vi "Test Pincer Ctrl.vi"() -> ()   [LabVIEW 2010]
uses:
  <vilib>/platform/TimedLoop/XDataNode/XDataNode.xnode
  <vilib>/Platform/TimedLoop/XDataNode/nitl_modes.ctl
  <vilib>/Platform/TimedLoop/XDataNode/XDNodeRunTimeDep.lvlib
  <vilib>/Platform/TimedLoop/XDataNode/wakeup.ctl
  <vilib>/Platform/TimedLoop/XDataNode/timing_clust.ctl
  <vilib>/rvi/interface/nirviReadWriteControl/nirviReadWriteControl.xnode
  FPGA Bitfiles/IRISSControl_FPGATarget_IRISSFPGAIOv3.3_r-h2UkgnQFc.lvbitx
  IRISS_FPGA_IO_v3.3.vi
  <vilib>/rvi/interface/nirviOpenFPGA/nirviOpenFPGA.xnode
  <vilib>/rvi/interface/nirviCloseFPGA/nirviCloseFPGA.xnode
  <vilib>/rvi/interface/nirviMethod/nirviMethod.xnode
panel:
  in  "Motion [%]":dbl min=0.0 max=1.0 step=0.05
  out "error out":errorcluster
  in  "stop":bool
  in  "Duty Limits [max,min]":dbl[](array[numeric])=[0.1, 0.05]
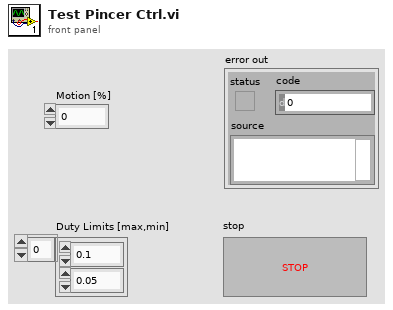
[diagram p1: front panel]
types:
  T1 = typedef "XDNodeRunTimeDep.lvlib/timing_clust.ctl" = cluster{"Expected End [f-1]":u64, "Actual End [f-1]":u64, "Finished Late? [f-1]":bool, "Expected End [i-1]":u64, "Actual End [i-1]":u64, "Finished Late? [i-1]":bool, "Expected Start [i]":u64, "Actual Start [i]":u64, "Expected Start [f]":u64, "Actual Start [f]":u64, "Source Name":string, "Structure Name":string, "Period":i64, "Deadline":i64, "Offset":i64, "Start":i64, "Priority":i32, "Timeout":i32, "Mode":T2, "Wakeup Reason":T3, "Error":errorcluster, "Source Type":string, "Secondary Source Type":string, "Global End Time":u64, "Global Start Time":u64, "Frame Duration":u64, "Iteration Duration":u64, "Assigned CPU":i32, "I/O Scan Engine Mode":u32}
  T2 = typedef "XDNodeRunTimeDep.lvlib/nitl_modes.ctl" = enum32{"No Change", "Process missed periods, maintain original phase", "Discard missed periods, maintain original phase", "Process missed periods, ignore original phase", "Discard missed periods, ignore original phase"}
  T3 = typedef "XDNodeRunTimeDep.lvlib/wakeup.ctl" = enum32{"Normal", "Aborted", "Asynchronous wakeup", "Timing source error", "Timed loop error", "Timeout"}
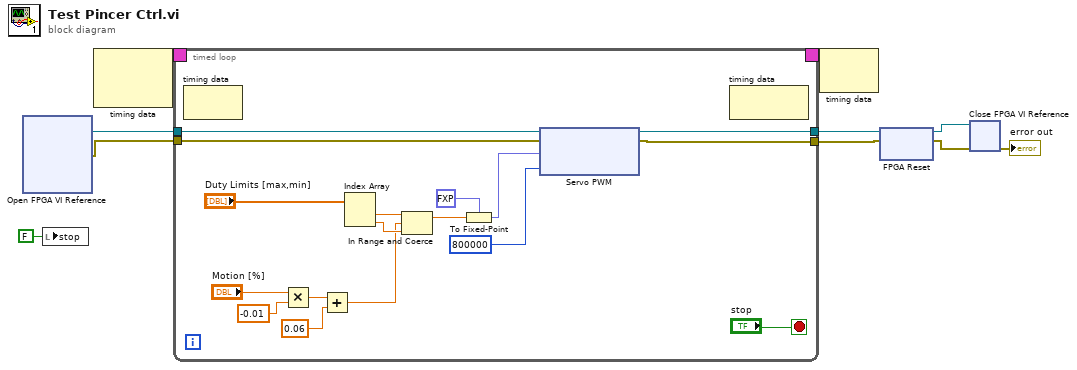
[diagram p0: block diagram]
diagram:
  n1 = xnode "Open FPGA VI Reference"() -> ("FPGA VI Reference Out"=w8:refnum<k20>, "error out"=w7:errorcluster)  [unwired: 2 in]
  n2 = local write "stop"(FALSE ("stop")) -> ()
  n3 = node-c288() -> (w10:T1)  [unwired: 2 in]
  n4 = timed-loop {
    timing: w10 -> [_]
    timing-out: [_] -> w9
    tunnel: w8 -> [w26]
    tunnel: w7 -> [w27]
    tunnel: [w18] -> w4
    tunnel: [w16] -> w2
    stop <- "stop" stop-if-true
    n5 = node-c288() -> ()  [unwired: 1 in, 1 out]
    n6 = Multiply(x="Motion [%]", y=-0.01) -> (x*y=w12:dbl)
    n7 = Add(x=w12, y=0.06) -> (x+y=w11:dbl)
    n8 = Index Array(array="Duty Limits [max,min]") -> (element #1=w25:dbl, element #2=w24:dbl)  [unwired: 2 in]
    n9 = In Range and Coerce(upper limit=w25, x=w11, lower limit=w24) -> (coerced(x)=w23:dbl)  [unwired: 1 out]
    n10 = To Fixed-Point(fixed-point type=fxp<+,32,0> 0.0 ("PWM1"), number=w23) -> (fixed-point=w19:fxp<+,32,0>)
    n11 = xnode "Servo PWM"("FPGA VI Reference In"=w26, "error in"=w27, "PWM1"=w19, "Period 1 (Ticks)"=u32 800000) -> ("FPGA VI Reference Out"=w18:refnum<k20>, "error out"=w16:errorcluster)
    n12 = node-c288() -> ()  [unwired: 1 in, 1 out]
  }
  n13 = node-c288(w9) -> ()  [unwired: 1 out]
  n14 = xnode "FPGA Reset"("FPGA VI Reference In"=w4, "error in"=w2) -> ("FPGA VI Reference Out"=w6:refnum<k20>, "error out"=w5:errorcluster)
  n15 = xnode "Close FPGA VI Reference"("FPGA VI Reference In"=w6, "error in"=w5) -> ("error out"=→"error out":errorcluster)
